vi "String_Type_Checker.vi"(11 "String":string) -> (3 "Type":string)   [LabVIEW 2025, in "Automotive Ethernet Bus Monitor UI.lvlib" / "Table_Filtering.lvlib"]
uses:
  Table_Filtering.lvlib
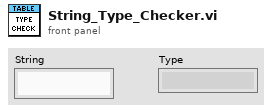
[diagram p1: front panel]
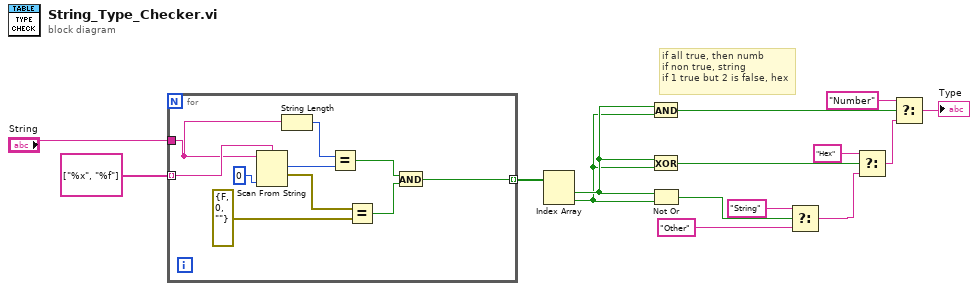
[diagram p0: block diagram]
diagram:
  # "if all true, then numb\nif non true, string\nif 1 true but 2 is false, hex"
  n1 = for {
    tunnel: string[] ["%x", "%f"] -> [w25] mode=indexing
    tunnel: "String" -> [w24]
    tunnel: [w17] -> w13 mode=indexing
    n2 = Scan From String(format string=w25, input string=w24, default 1=0 ("length")) -> (offset past scan=w23:u32, error out=w20:errorcluster)  [unwired: 3 in, 1 out]
    n3 = String Length(string=w24) -> (length=w22:i32)
    n4 = Equal?(x=w22, y=w23) -> (x = y?=w19:bool)
    n5 = Equal?(x=w20, y=errorcluster {"status"=FALSE, "code"=0, "source"=""} ("error constant")) -> (x = y?=w18:bool)
    n6 = And(x=w19, y=w18) -> (x .and. y?=w17:bool)
  }
  n7 = Index Array(array=w13) -> (element #1=w3:bool, element #2=w2:bool)  [unwired: 2 in]
  n8 = And(x=w3, y=w2) -> (x .and. y?=w6:bool)
  n9 = Exclusive Or(1:w2, 2:w3) -> (0:w11:bool)
  n10 = Not Or(1:w2, 2:w3) -> (0:w10:bool)
  n11 = Select(t="String", s=w10, f="Other") -> (s? t:f=w9:string)
  n12 = Select(t="Hex", s=w11, f=w9) -> (s? t:f=w7:string)
  n13 = Select(t="Number", s=w6, f=w7) -> (s? t:f=→"Type":string)
